vi "Read Status.vi"(8 "error in (no error)":errorcluster, 11 "MotorDrive in":refnum<class "MotorDrive.lvclass">) -> (0 "error out":errorcluster, 2 "Status":T1, 3 "MotorDrive out":refnum<class "MotorDrive.lvclass">)   [LabVIEW 2016, in "MotorDrive.lvclass"]
uses:
  MotorDrive.lvclass
  Globals/Status--cluster.ctl
  MotorDrive.lvclass/MotorDrive.ctl
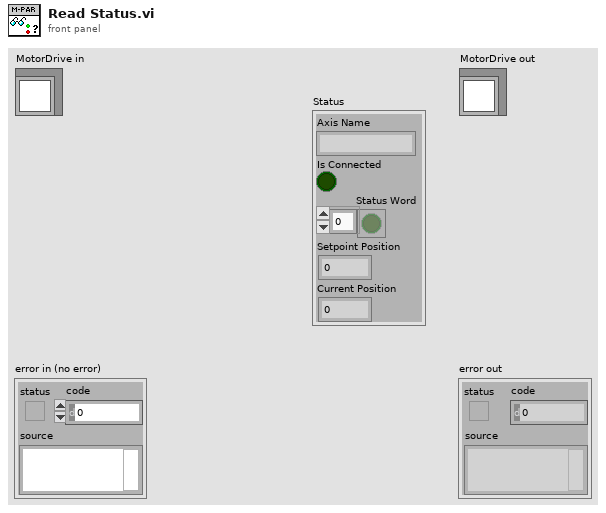
[diagram p1: front panel]
types:
  T1 = typedef "MotorDrive.lvclass/Status--cluster.ctl" = cluster{"Axis Name":string, "Is Connected":bool, "Status Word":bool[], "Setpoint Position":dbl, "Current Position":dbl}
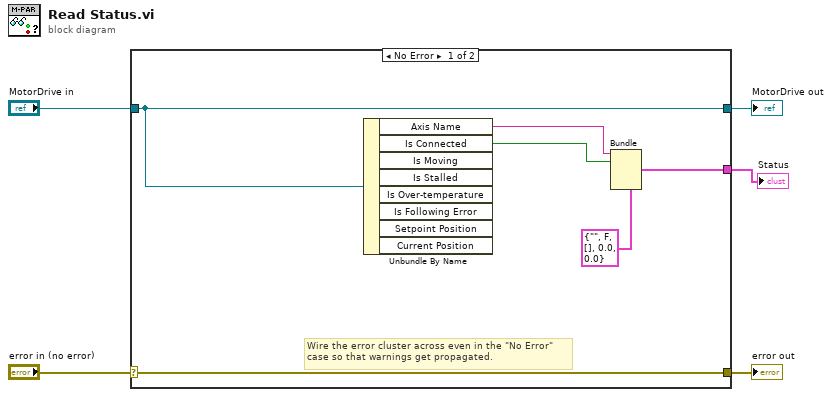
[diagram p0: block diagram]
diagram:
  n1 = case shown="No Error" "error in (no error)" {
    selector: "error in (no error)" -> [w11 w13]
    tunnel: [w11 w13] -> w4
    tunnel: [w10 w12] -> w2
    tunnel: "MotorDrive in" -> [w10 w12]
    tunnel: [w6 _] -> w1
    frame No Error {
      # "Wire the error cluster across even in the \"No Error\"\ncase so that warnings get propagated."
      n2 = Unbundle By Name(w10) -> ("Axis Name"=w9:string, "Is Connected"=w8:bool)  [unwired: 6 out]
      n3 = Bundle(cluster=T1 {"Axis Name"="", "Is Connected"=FALSE, "Status Word"=[], "Setpoint Position"=0.0, "Current Position"=0.0} ("Stauts"), "Axis Name"=w9, "Is Connected"=w8) -> (w6:T1)  [unwired: 3 in]
    }
    frame Error {
    }
  }
  "error out" <- w4
  "MotorDrive out" <- w2
  "Status" <- w1
